vi "Write Data.vi"(8 "error in (no error)":errorcluster, 11 "DbMeasurement in 2":refnum<class "DbMeasurement.lvclass">) -> (0 "error out":errorcluster, 3 "DbMeasurement out 2":refnum<class "DbMeasurement.lvclass">)   [LabVIEW 2013, in "DbMeasurement.lvclass"]
doc: "This dynamic dispatch method should be overwritten to write data to a file using whatever data writing technique desired."
uses:
  DbMeasurement.lvclass
  DbMeasurement.lvclass/DbMeasurement.ctl
  <vilib>/addons/database/NI_Database_API.lvlib
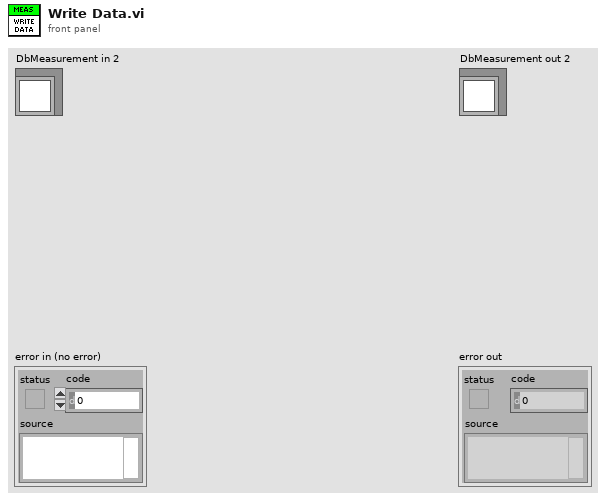
[diagram p1: front panel]
types:
  T1 = typedef "NI_Database_API.lvlib/Conn ObjectReference.ctl" = refnum<k1>
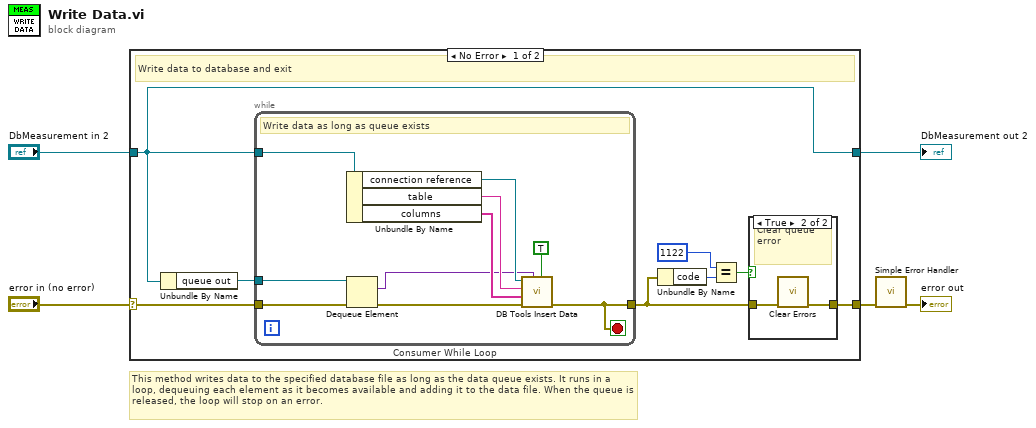
[diagram p0: block diagram]
diagram:
  # "This method writes data to the specified database file as long as the data queue exists. It runs in a loop, dequeuing each element as it becomes available and adding it to the data file. When the queue is released, the loop will stop on an error."
  n1 = case shown="No Error" "error in (no error)" {
    selector: "error in (no error)" -> [w13 w27]
    tunnel: "DbMeasurement in 2" -> [w10 w28]
    tunnel: [w10 w28] -> w2
    tunnel: [w11 w27] -> w4
    frame No Error {
      # "Write data to database and exit"
      n2 = Unbundle By Name(w10) -> ("queue out"=w12:refnum<queue>)
      n3 = while "Consumer While Loop" {
        tunnel: w10 -> [w26]
        tunnel: w13 -> [w21]
        tunnel: [w20] -> w9
        tunnel: w12 -> [w18]
        stop <- w20 stop-if-true
        # "Write data as long as queue exists"
        n4 = Unbundle By Name(w26) -> ("connection reference"=w22:T1, "table"=w24:string, "columns"=w25:string[])
        n5 = Dequeue Element(queue=w18, error in (no error)=w21) -> (element=w17:variant, error out=w19:errorcluster)  [unwired: 1 in, 2 out]
        n6 = call <vilib>:"DB Tools Insert Data.vi"("create table? (F)"=TRUE, "data"=w17, "error in (no error)"=w19, "columns"=w25, "table"=w24, "connection reference"=w22) -> ("error out"=w20:errorcluster)  [unwired: 4 in, 1 out]
      }
      n7 = Unbundle By Name(w9) -> ("code"=w8:i32)
      n8 = Equal?(x=1122, y=w8) -> (x = y?=w6:bool)
      n9 = case shown="True" w6 {
        tunnel: [w14 w16] -> w11
        tunnel: w9 -> [w14 w15]
        frame False {
          # "Keep errors"
        }
        frame True {
          # "Clear queue error"
          n10 = call <vilib>:"Clear Errors.vi"("error in (no error)"=w15) -> ("error out"=w16:errorcluster)  [unwired: 6 in]
        }
      }
    }
    frame Error {
      # "Pass through and exit"
    }
  }
  "DbMeasurement out 2" <- w2
  n11 = call <vilib>:"Simple Error Handler.vi"("error in (no error)"=w4) -> ("error out"=→"error out":errorcluster)  [unwired: 4 in, 4 out]
